vi "Collect All Measurements.vi"(0 "Rigid Connection":bool, 4 "Limits":T8[](array[typedef]), 6 "Connection Offsets":T1[](array[typedef]), 7 "Position":T7[](array[typedef]), 8 "Type":T6[](array[typedef]), 9 "Actuator Meas. Disp & Forces":dbl[][](array[numeric]), 10 "Cmd In":T10[](array[typedef]), 11 "Within Limits In":T2[](array[typedef])) -> (1 "Within Limits Out":T2[](array[typedef]), 3 "Measurements Out":T11[](array[typedef]), 5 "Cmds Out":T10[](array[typedef]))   [LabVIEW 2009]
uses:
  Limits/Within Limits Matrix.ctl
  Limits/Actuator Faults.ctl
  Limits/Cart Force Faults.ctl
  Limits/Cart Disp Faults.ctl
  Measurements.ctl
  Act & Cart Commands.ctl
  Limit Settings.ctl
  Limit Matrix.ctl
  Data Access Objects/Metadata/LBCB Position.ctl
  Data Access Objects/Metadata/LBCB Type.ctl
  Data Access Objects/Offsets/Connection Offsets.ctl
  Data Access Objects/Metadata/LBCB Number.ctl
panel:
  # "(inch)"
  # "X"
  # "(inch)"
  # "Y"
  # "(inch)"
  # "Z"
  # "Xglobal = T*Xlocal"
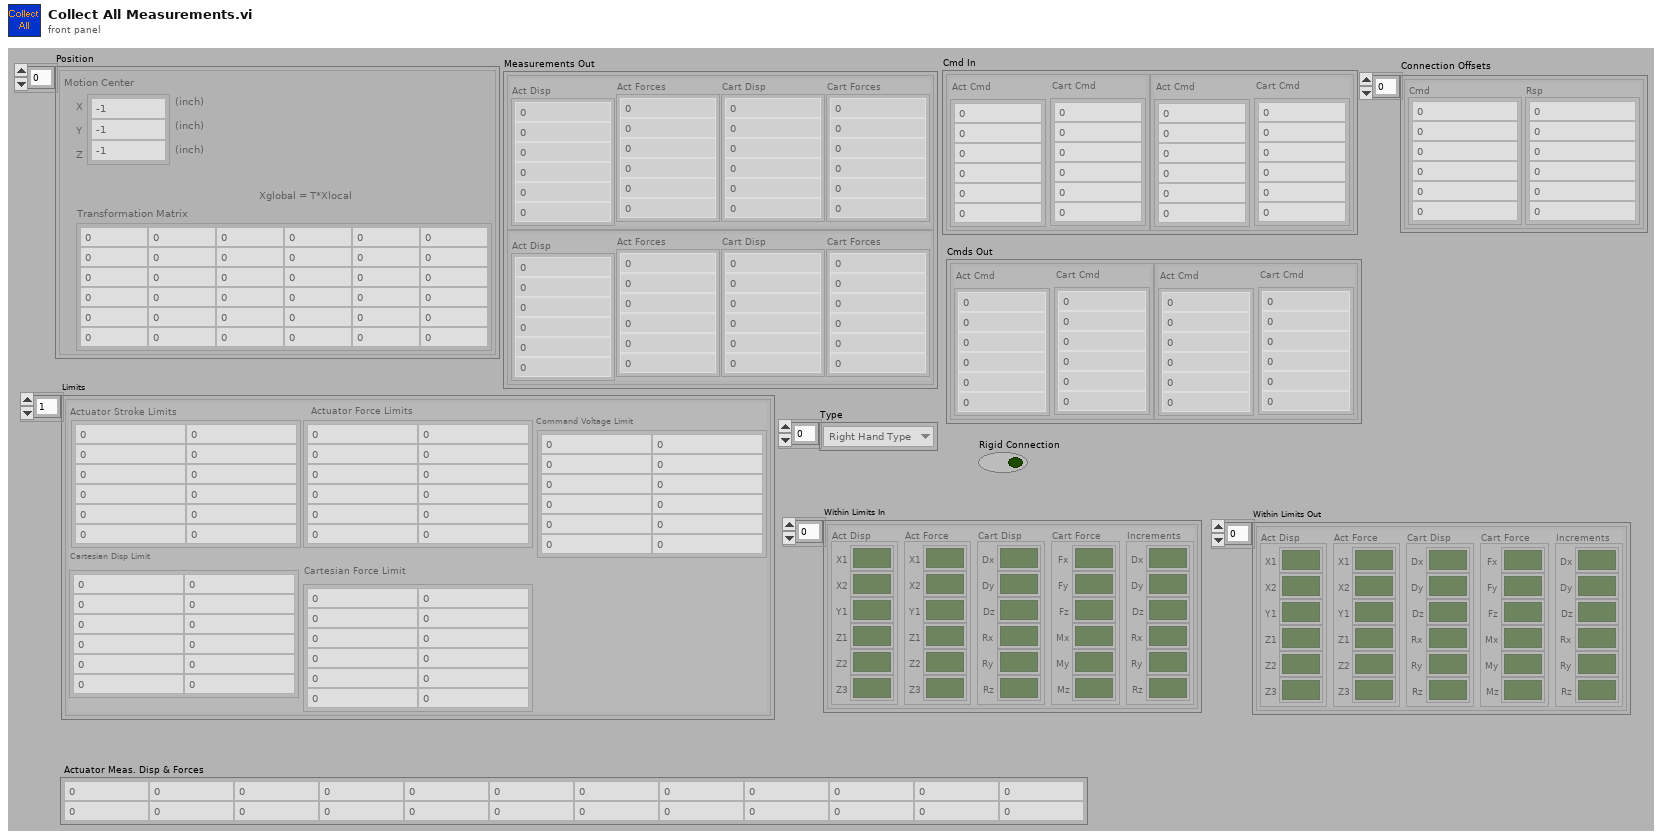
[diagram p1: front panel]
types:
  T1 = typedef "Connection Offsets.ctl" = cluster{"Cmd":dbl[], "Rsp":dbl[]}
  T2 = typedef "Within Limits Matrix.ctl" = cluster{"Act Disp":T3, "Act Force":T3, "Cart Force":T4, "Cart Disp":T5, "Increments":T5}
  T3 = typedef "Actuator Faults.ctl" = cluster{"X1":bool, "X2":bool, "Y1":bool, "Z1":bool, "Z2":bool, "Z3":bool}
  T4 = typedef "Cart Force Faults.ctl" = cluster{"Fx":bool, "Fy":bool, "Fz":bool, "Mx":bool, "My":bool, "Mz":bool}
  T5 = typedef "Cart Disp Faults.ctl" = cluster{"Dx":bool, "Dy":bool, "Dz":bool, "Rx":bool, "Ry":bool, "Rz":bool}
  T6 = typedef "LBCB Type.ctl" = enum16{"Right Hand Type", "Left Hand Type"}
  T7 = typedef "LBCB Position.ctl" = cluster{"Motion Center":dbl[], "Transformation Matrix":dbl[][]}
  T8 = typedef "Limit Settings.ctl" = cluster{"Actuator Force Limits":T9, "Actuator Stroke Limits":T9, "Cartesian Disp Limit":T9, "Cartesian Force Limit":T9, "Command Voltage Limit":T9}
  T9 = typedef "Limit Matrix.ctl" = dbl[][]
  T10 = typedef "Act & Cart Commands.ctl" = cluster{"Act Cmd":dbl[], "Cart Cmd":dbl[]}
  T11 = typedef "Measurements.ctl" = cluster{"Act Disp":dbl[], "Act Forces":dbl[], "Cart Disp":dbl[], "Cart Forces":dbl[]}
  T12 = typedef "LBCB Number.ctl" = enum16{"LBCB1", "LBCB2"}
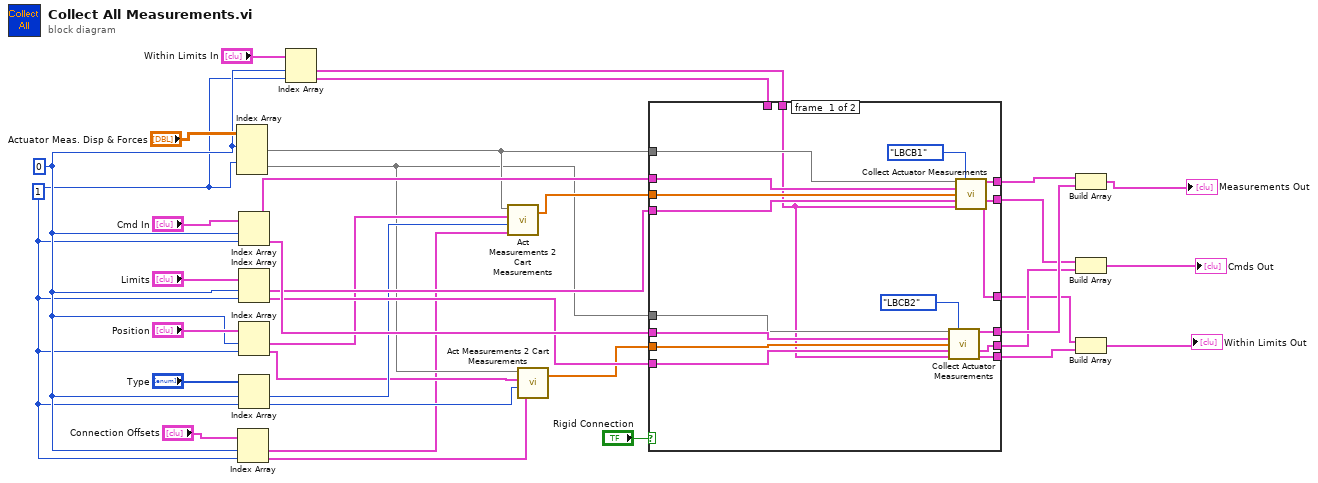
[diagram p0: block diagram]
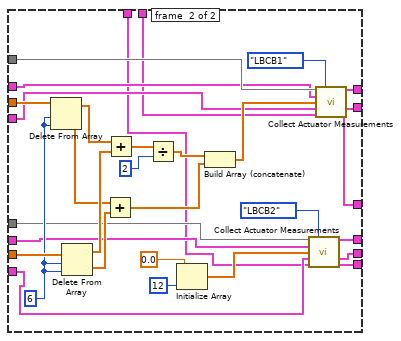
[diagram p2: hidden frame]
diagram:
  w3 = 1 ("index (row)")
  w4 = 0 ("index (row)")
  n1 = Index Array(array="Actuator Meas. Disp & Forces", index (row) #1=w4, index (row) #2=w3) -> (element #1=w18:dbl[], element #2=w14:dbl[])  [unwired: 2 in]
  n2 = Index Array(array="Connection Offsets", index #1=w4, index #2=w3) -> (element #1=w2:T1, element #2=w1:T1)
  n3 = Index Array(array="Cmd In", index #1=w4, index #2=w3) -> (element #1=w29:T10, element #2=w30:T10)
  n4 = Index Array(array="Limits", index #1=w4, index #2=w3) -> (element #1=w28:T8, element #2=w27:T8)
  n5 = Index Array(array="Position", index #1=w4, index #2=w3) -> (element #1=w16:T7, element #2=w11:T7)
  n6 = Index Array(array="Type", index #1=w4, index #2=w3) -> (element #1=w17:T6, element #2=w12:T6)
  n7 = Index Array(array="Within Limits In", index #1=w4, index #2=w3) -> (element #1=w7:T2, element #2=w6:T2)
  n8 = call "Act Measurements 2 Cart Measurements.vi"("Connection Offsets"=w2, "Type"=w17, "LBCB Position"=w16, "Actuator Meas. \nDisp & Forces"=w18) -> ("Cart Measured\nDisp & Forces"=w15:dbl[])  [unwired: 1 in]
  n9 = call "Act Measurements 2 Cart Measurements.vi"("Connection Offsets"=w1, "Type"=w12, "LBCB Position"=w11, "Actuator Meas. \nDisp & Forces"=w14) -> ("Cart Measured\nDisp & Forces"=w13:dbl[])  [unwired: 1 in]
  n10 = case shown="False" "Rigid Connection" {
    tunnel: w30 -> [w50 w59]
    tunnel: w29 -> [w49 w62]
    tunnel: w28 -> [w48 w61]
    tunnel: w27 -> [w47 w58]
    tunnel: [w46 w81] -> w26
    tunnel: [w45 w80] -> w25
    tunnel: [w44 w79] -> w23
    tunnel: [w43 w78] -> w22
    tunnel: [w42 w77] -> w20
    tunnel: [w41 w76] -> w19
    tunnel: w18 -> [w40 w63]
    tunnel: w15 -> [w39 w73]
    tunnel: w14 -> [w38 w60]
    tunnel: w13 -> [w37 w75]
    tunnel: w7 -> [w36 w54]
    tunnel: w6 -> [_ w53]
    frame #0 {
      n11 = call "Collect Actuator Measurements.vi"("Actuator Meas. \nDisp & Forces"=w38, "LBCB Number"=LBCB_Number."LBCB2", "Commands In"=w50, "Cartesian Meas. \nDisp & Forces"=w37, "Limits"=w47, "Within Limits In"=w36) -> ("Measurements Out"=w45:T11, "Commands Out"=w43:T10, "Within Limits Out"=w41:T2)  [unwired: 4 in, 3 out]
      n12 = call "Collect Actuator Measurements.vi"("Actuator Meas. \nDisp & Forces"=w40, "LBCB Number"=LBCB_Number."LBCB1", "Commands In"=w49, "Cartesian Meas. \nDisp & Forces"=w39, "Limits"=w48, "Within Limits In"=w36) -> ("Measurements Out"=w46:T11, "Commands Out"=w44:T10, "Within Limits Out"=w42:T2)  [unwired: 4 in, 3 out]
    }
    frame #1 {
      w74 = 6 ("index")
      n13 = Delete From Array(array=w73, length=w74, index=w74) -> (deleted portion=w69:dbl[], array with subset deleted=w71:dbl[])
      n14 = Delete From Array(array=w75, length=w74, index=w74) -> (deleted portion=w68:dbl[], array with subset deleted=w70:dbl[])
      n15 = Add(x=w69, y=w68) -> (x+y=w65:dbl[])
      n16 = Add(x=w71, y=w70) -> (x+y=w72:dbl[])
      n17 = Divide(x=w72, y=2) -> (x/y=w66:dbl[])
      n18 = Initialize Array(0.0 ("element"), 12 ("dimension size")) -> (w55:dbl[])
      n19 = Build Array (concatenate)(w66, w65) -> (w64:dbl[])
      n20 = call "Collect Actuator Measurements.vi"("Actuator Meas. \nDisp & Forces"=w60, "LBCB Number"=LBCB_Number."LBCB2", "Commands In"=w59, "Cartesian Meas. \nDisp & Forces"=w55, "Limits"=w58, "Within Limits In"=w53) -> ("Measurements Out"=w80:T11, "Commands Out"=w78:T10, "Within Limits Out"=w76:T2)  [unwired: 4 in, 3 out]
      n21 = call "Collect Actuator Measurements.vi"("Actuator Meas. \nDisp & Forces"=w63, "LBCB Number"=LBCB_Number."LBCB1", "Commands In"=w62, "Cartesian Meas. \nDisp & Forces"=w64, "Limits"=w61, "Within Limits In"=w54) -> ("Measurements Out"=w81:T11, "Commands Out"=w79:T10, "Within Limits Out"=w77:T2)  [unwired: 4 in, 3 out]
    }
  }
  n22 = Build Array(w26, w25) -> (→"Measurements Out":T11[])
  n23 = Build Array(w23, w22) -> (→"Cmds Out":T10[])
  n24 = Build Array(w20, w19) -> (→"Within Limits Out":T2[])
